vi "Open Solver.vi"(8 "error in (no error)":errorcluster, 11 "Solver Path":path) -> (0 "error IO":errorcluster, 3 "Solver VI":T1)   [LabVIEW 2024, in "Word Search Scorer.lvlib"]
uses:
  Word Search Scorer.lvlib
  Solver VI Ref Type.ctl
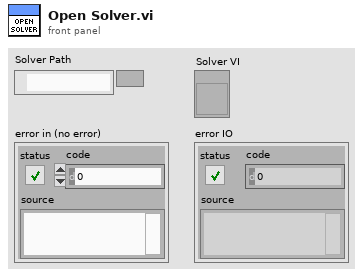
[diagram p1: front panel]
types:
  T1 = typedef "Word Search Scorer.lvlib/Solver VI Ref Type.ctl" = refnum<vi>
  T2 = enum32{"Invalid", "Standard", "Closed", "Hidden", "Minimized", "Maximized"}
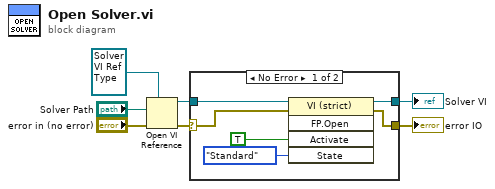
[diagram p0: block diagram]
diagram:
  n1 = Open VI Reference(type specifier VI Refnum (for type only)=T1 refnum ("Solver VI"), vi path="Solver Path", error in (no error)="error in (no error)") -> (vi reference=w5:T1, error out=w6:errorcluster)  [unwired: 3 in]
  n2 = case shown="No Error" w6 {
    selector: w6 -> [w9 w15]
    tunnel: w5 -> [w13 w14]
    tunnel: [w8 w15] -> w3
    tunnel: [w10 w14] -> w1
    frame No Error {
      n3 = invoke class="VI (strict)" method="FP.Open"(reference=w13, error in=w9, "Activate"=TRUE ("Activate?"), "State"=T2."Standard") -> (reference out=w10:T1, error out=w8:errorcluster)  [unwired: 1 in, 3 out]
    }
    frame Error {
    }
  }
  "Solver VI" <- w1
  "error IO" <- w3
